vi "Log.vi"(8 "error in (no error)":errorcluster, 10 "Log Text":string, 11 "Queue Sink in":refnum<class "Queue Sink.lvclass">) -> (0 "error out":errorcluster, 3 "Queue Sink out":refnum<class "Queue Sink.lvclass">)   [LabVIEW 2020, in "LV Log.lvlib" / "Queue Sink.lvclass"]
uses:
  Queue Sink.lvclass
  Queue Sink.lvclass/Queue Sink.ctl
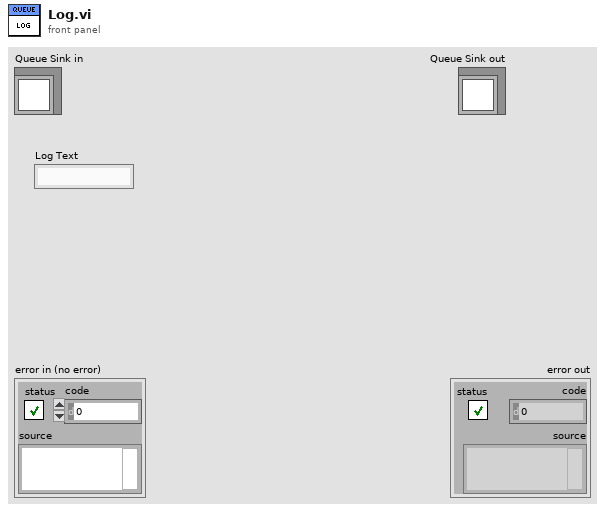
[diagram p1: front panel]
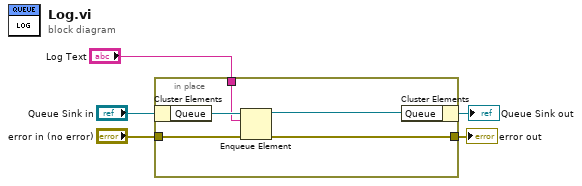
[diagram p0: block diagram]
diagram:
  n1 = in-place {
    in-place-border: "Log Text" -> [w8]
    in-place-border: "error in (no error)" -> [w7]
    in-place-border: [w6] -> w3
    n2 = in-place-cluster #1("Queue Sink in") -> ("Queue"=w10:refnum<queue>)
    n3 = Enqueue Element(queue=w10, element=w8, error in (no error)=w7) -> (queue out=w9:refnum<queue>, error out=w6:errorcluster)  [unwired: 1 in, 1 out]
    n4 = in-place-cluster #1("Queue"=w9) -> (→"Queue Sink out":refnum<class "Queue Sink.lvclass">)
  }
  "error out" <- w3
